vi "Initilize driver.vi"(8 "error in":errorcluster, 10 "input settings":T1={"LeCroy IP"="169.254.20.90", "Ch1"={"On/Off"=FALSE, "Bandwidth (Dropdown)"=0, "Vertical Range (V)"=5000.0, "Vertical Offset (V)"=0.0}, "Ch2"={"On/Off"=FALSE, "Bandwidth (Dropdown)"=0, "Vertical Range (V)"=0.2, "Vertical Offset (V)"=0.0}, "Ch3"={"On/Off"=TRUE, "Bandwidth (Dropdown)"=0, "Vertical Range (V)"=1.2, "Vertical Offset (V)"=0.0}, "Ch4"={"On/Off"=TRUE, "Bandwidth (Dropdown)"=0, "Vertical Range (V)"=0.2, "Vertical Offset (V)"=0.0}, "T axis"={"Time base (s/div)"=0.0002, "Time offset (s)"=0.0, "Max Sample Points"=0}, "Trig"={"Trigger mode"=2, "Trigger Slope"=0, "Trigger Source"=1, "Trigger Level (V)"=0.04}, "Timeout (ms)"=0.0} caption="Settings" {"Trig"."Trigger mode" items=["Auto", "Normal", "Single", "Single, auto trigger"]; "Trig"."Trigger Slope" items=["Rising", "Falling"]; "Trig"."Trigger Source" items=["Channel 1", "Channel 2", "Channel 3", "Channel 4", "External", "Power Line"]; "Trig"."Trigger Level (V)" format="%#_6p"; "T axis"."Max Sample Points" format="%.0p" items=["50"=50, "100"=100, "250"=250, "500"=500, "1000"=1000, "2500"=2500, "5K"=5000, "10K"=10000, "25K"=25000, "50K"=50000, "100K"=100000, "250K"=250000, "500K"=500000, "1M"=1000000, "2M"=2000000, "2.5M"=2500000, "5M"=5000000, "10M"=10000000, "25M"=25000000, "50M"=50000000, "100M"=100000000]; "T axis"."Time base (s/div)" format="%#_6p"; "Ch4"."Bandwidth (Dropdown)" items=["Full", "20MHZ", "25MHZ", "200MHZ", "250MHZ", "1GHZ", "3GHZ", "4GHZ"]; "Ch3"."Bandwidth (Dropdown)" items=["Full", "20MHZ", "25MHZ", "200MHZ", "250MHZ", "1GHZ", "3GHZ", "4GHZ"]; "Ch2"."Bandwidth (Dropdown)" items=["Full", "20MHZ", "25MHZ", "200MHZ", "250MHZ", "1GHZ", "3GHZ", "4GHZ"]; "Ch1"."Bandwidth (Dropdown)" items=["Full", "20MHZ", "25MHZ", "200MHZ", "250MHZ", "1GHZ", "3GHZ", "4GHZ"]}) -> (0 "error out":errorcluster, 2 "output settings":T1={"LeCroy IP"="169.254.20.90", "Ch1"={"On/Off"=FALSE, "Bandwidth (Dropdown)"=0, "Vertical Range (V)"=5000.0, "Vertical Offset (V)"=0.0}, "Ch2"={"On/Off"=FALSE, "Bandwidth (Dropdown)"=0, "Vertical Range (V)"=0.2, "Vertical Offset (V)"=0.0}, "Ch3"={"On/Off"=TRUE, "Bandwidth (Dropdown)"=0, "Vertical Range (V)"=1.2, "Vertical Offset (V)"=0.0}, "Ch4"={"On/Off"=TRUE, "Bandwidth (Dropdown)"=0, "Vertical Range (V)"=0.2, "Vertical Offset (V)"=0.0}, "T axis"={"Time base (s/div)"=0.0002, "Time offset (s)"=0.0, "Max Sample Points"=0}, "Trig"={"Trigger mode"=2, "Trigger Slope"=0, "Trigger Source"=1, "Trigger Level (V)"=0.04}, "Timeout (ms)"=0.0} caption="Settings" {"Trig"."Trigger mode" items=["Auto", "Normal", "Single", "Single, auto trigger"]; "Trig"."Trigger Slope" items=["Rising", "Falling"]; "Trig"."Trigger Source" items=["Channel 1", "Channel 2", "Channel 3", "Channel 4", "External", "Power Line"]; "Trig"."Trigger Level (V)" format="%#_6p"; "T axis"."Max Sample Points" format="%.0p" items=["50"=50, "100"=100, "250"=250, "500"=500, "1000"=1000, "2500"=2500, "5K"=5000, "10K"=10000, "25K"=25000, "50K"=50000, "100K"=100000, "250K"=250000, "500K"=500000, "1M"=1000000, "2M"=2000000, "2.5M"=2500000, "5M"=5000000, "10M"=10000000, "25M"=25000000, "50M"=50000000, "100M"=100000000]; "T axis"."Time base (s/div)" format="%#_6p"; "Ch4"."Bandwidth (Dropdown)" items=["Full", "20MHZ", "25MHZ", "200MHZ", "250MHZ", "1GHZ", "3GHZ", "4GHZ"]; "Ch3"."Bandwidth (Dropdown)" items=["Full", "20MHZ", "25MHZ", "200MHZ", "250MHZ", "1GHZ", "3GHZ", "4GHZ"]; "Ch2"."Bandwidth (Dropdown)" items=["Full", "20MHZ", "25MHZ", "200MHZ", "250MHZ", "1GHZ", "3GHZ", "4GHZ"]; "Ch1"."Bandwidth (Dropdown)" items=["Full", "20MHZ", "25MHZ", "200MHZ", "250MHZ", "1GHZ", "3GHZ", "4GHZ"]}, 3 "VISA resource name out":refnum<visa-resource-name>)   [LabVIEW 2013]
uses:
  Settings_TypeDef.ctl
  LeCroy Wave Series.lvlib
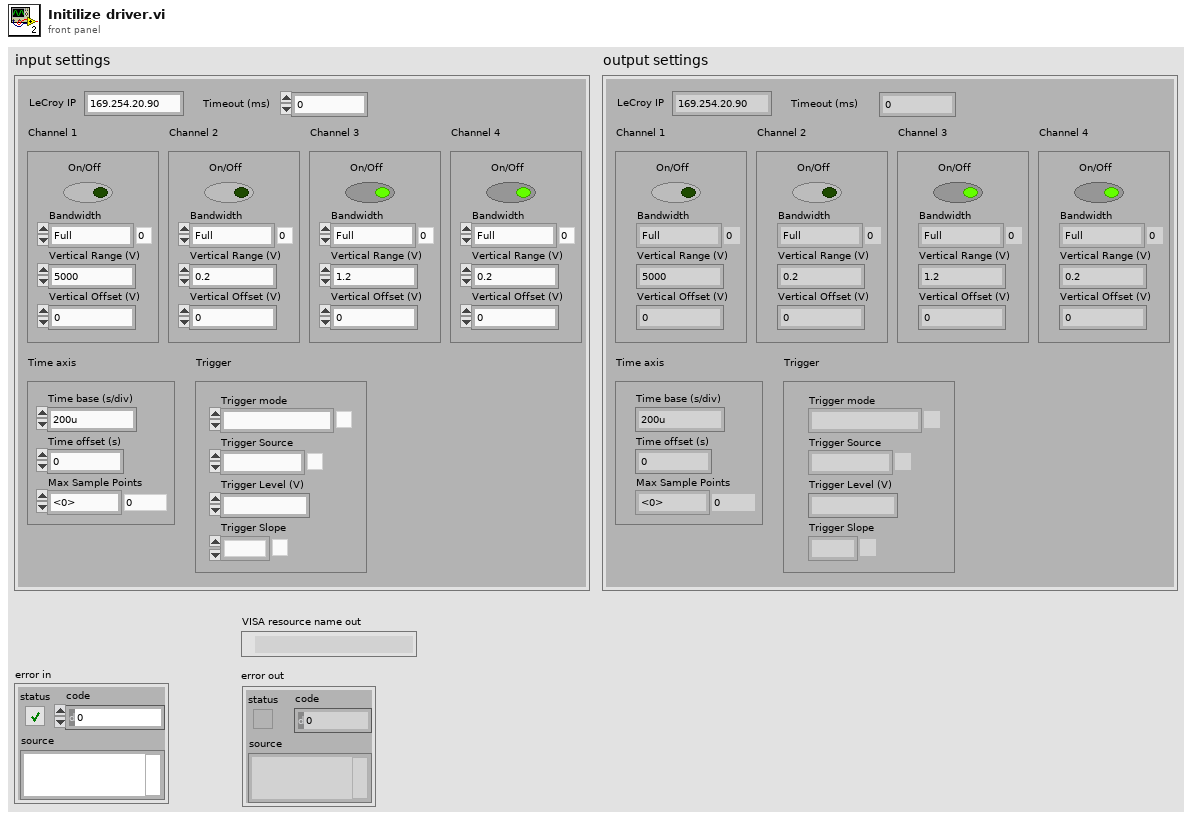
[diagram p1: front panel]
types:
  T1 = typedef "Settings_TypeDef.ctl" = cluster{"LeCroy IP":string, "Ch1":cluster{"On/Off":bool, "Bandwidth (Dropdown)":u16, "Vertical Range (V)":dbl, "Vertical Offset (V)":dbl}, "Ch2":cluster{"On/Off":bool, "Bandwidth (Dropdown)":u16, "Vertical Range (V)":dbl, "Vertical Offset (V)":dbl}, "Ch3":cluster{"On/Off":bool, "Bandwidth (Dropdown)":u16, "Vertical Range (V)":dbl, "Vertical Offset (V)":dbl}, "Ch4":cluster{"On/Off":bool, "Bandwidth (Dropdown)":u16, "Vertical Range (V)":dbl, "Vertical Offset (V)":dbl}, "T axis":cluster{"Time base (s/div)":dbl, "Time offset (s)":dbl, "Max Sample Points":i32}, "Trig":cluster{"Trigger mode":u16, "Trigger Slope":u16, "Trigger Source":u16, "Trigger Level (V)":dbl}, "Timeout (ms)":dbl}
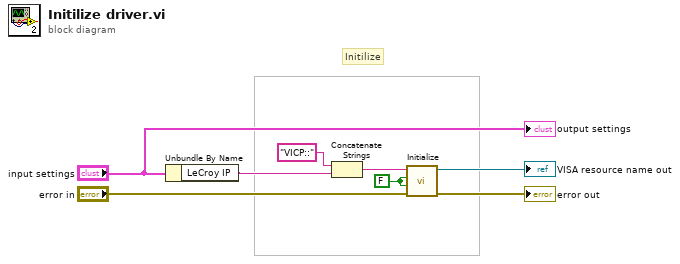
[diagram p0: block diagram]
diagram:
  w8 = FALSE ("Reset? (T: Yes)")
  # "Initilize"
  n1 = Unbundle By Name("input settings") -> ("LeCroy IP"=w4:string)
  n2 = Concatenate Strings("VICP::", w4) -> (w6:string)
  n3 = call "Initialize.vi"("error in (no error)"="error in", "Reset? (T: Yes)"=w8, "ID Query? (T: Yes)"=w8, "VISA resource name"=w6) -> ("error out"=→"error out":errorcluster, "VISA resource name out"=→"VISA resource name out":refnum<visa-resource-name>)  [unwired: 6 in]
  "output settings" <- "input settings"
